vi "LitePoint_GPRF_VSA_ReceivedPower_DataConversion.vi"(11 "read buffer":string="0,#14…ù-Á\n") -> (3 "value":sgl=3.0 format="%.2f")   [LabVIEW 2020, in "LitePoints.lvlib"]
uses:
  LitePoints.lvlib
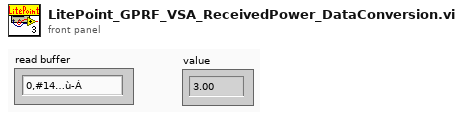
[diagram p1: front panel]
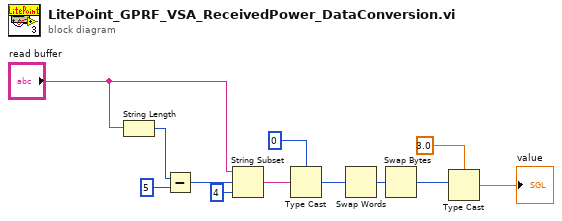
[diagram p0: block diagram]
diagram:
  n1 = String Length(string="read buffer") -> (length=w4:i32)
  n2 = Subtract(x=w4, y=5) -> (x-y=w2:i32)
  n3 = String Subset(string="read buffer", offset (0)=w2, length (rest)=4 ("length (rest)")) -> (substring=w6:string)
  n4 = Type Cast(type=u32 0, x=w6) -> (*(type *) &x=w11:u32)
  n5 = Swap Words(1:w11) -> (0:w10:u32)
  n6 = Swap Bytes(anything=w10) -> (byte swapped=w9:u32)
  n7 = Type Cast(type=sgl 3.0, x=w9) -> (*(type *) &x=→"value":sgl)
